vi "Plug_in_Directories.vi"() -> (2 "Trav_Profile_Plug_Ins":path, 3 "Initial":path, 4 "Pre_Analysis_Plugins":path, 5 "Per Block":path, 6 "Final":path)   [LabVIEW 2016]
uses:
  Globals/Constants_global.vi
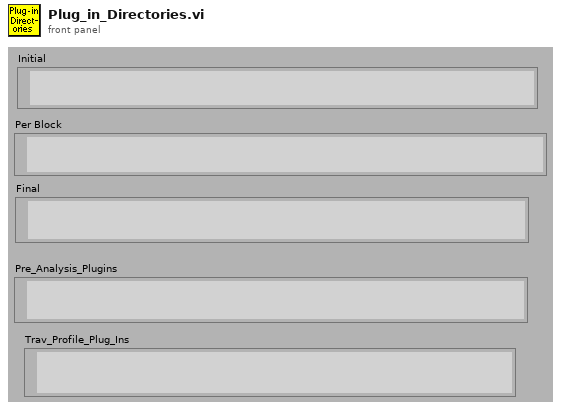
[diagram p1: front panel]
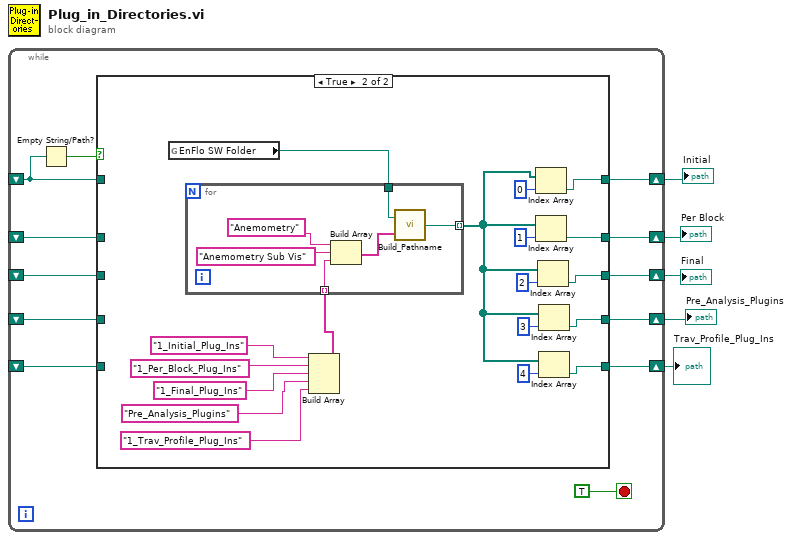
[diagram p0: block diagram]
diagram:
  n1 = while {
    shift-right: [w15] -> w3
    shift-left: _ -> [w12]
    shift-right: [w14] -> w4
    shift-left: _ -> [w11]
    shift-right: [w13] -> w5
    shift-left: _ -> [w10]
    shift-right: [w9] -> w2
    shift-left: _ -> [w8]
    shift-right: [w7] -> w1
    shift-left: _ -> [w6]
    stop <- TRUE stop-if-true
    n2 = Empty String/Path?(string/path=w12) -> (empty?=w16:bool)
    n3 = case shown="True" w16 {
      tunnel: [w22 w32] -> w15
      tunnel: [w21 w31] -> w14
      tunnel: [w20 w30] -> w13
      tunnel: w12 -> [w22 _]
      tunnel: w11 -> [w21 _]
      tunnel: w10 -> [w20 _]
      tunnel: [w19 w28] -> w9
      tunnel: w8 -> [w19 _]
      tunnel: [w18 w25] -> w7
      tunnel: w6 -> [w18 _]
      frame False {
      }
      frame True {
        n4 = global read "Constants_global.vi" "EnFlo SW Folder"() -> (w37:path)
        n5 = Build Array("1_Initial_Plug_Ins", "1_Per_Block_Plug_Ins", "1_Final_Plug_Ins", "Pre_Analysis_Plugins", "1_Trav_Profile_Plug_Ins") -> (w36:string[])
        n6 = for {
          tunnel: w37 -> [w43]
          tunnel: w36 -> [w42] mode=indexing
          tunnel: [w41] -> w24 mode=indexing
          n7 = Build Array("Anemometry", "Anemometry Sub Vis", w42) -> (w46:string[])
          n8 = call "Build_Pathname.vi"("PathElements"=w46, "PathnameIn"=w43) -> ("AppendedPath"=w41:path)
        }
        n9 = Index Array(array=w24, index=0) -> (element=w32:path)
        n10 = Index Array(array=w24, index=1) -> (element=w31:path)
        n11 = Index Array(array=w24, index=2) -> (element=w30:path)
        n12 = Index Array(array=w24, index=3) -> (element=w28:path)
        n13 = Index Array(array=w24, index=4) -> (element=w25:path)
      }
    }
  }
  "Initial" <- w3
  "Final" <- w5
  "Per Block" <- w4
  "Pre_Analysis_Plugins" <- w2
  "Trav_Profile_Plug_Ins" <- w1
